vi "verifySignatureExample.vi"(8 "error in (no error)":errorcluster, 10 "verifySignatureRequestid":dbl) -> (0 "error out":errorcluster, 2 "verifySignatureResponse":T3)   [LabVIEW 2014]
uses:
  Type Defs/verifySignatureResponse.ctl
  Type Defs/generateIntegersRequest.ctl
  Type Defs/generateSignedIntegersResponse.ctl
  Sub Vi's/verifySignatures/verifySignatureIntegers.vi
  Random JSON API.lvlib
panel:
  in  "Force verification failure":bool
  out "Response":T1={"result"={"random"={"method"="", "hashedApiKey"="", "n"=0, "min"=0, "max"=0, "replacement"=TRUE, "base"=10, "data"=[], "completionTime"="", "serialNumber"=0}, "signature"="", "bitsUsed"=0, "bitsLeft"=0, "requestsLeft"=0, "advisoryDelay"=0}, "id"=0.0} {"result"."random"."base" items=["2"=2, "8"=8, "10"=10, "16"=16]}
  in  "Parameters":T2={"params"={"apiKey"="", "n"=0, "min"=0, "max"=0, "replacement"=TRUE, "base"=10}, "id"=0.0} {"params"."base" items=["2"=2, "8"=8, "10"=10, "16"=16]}
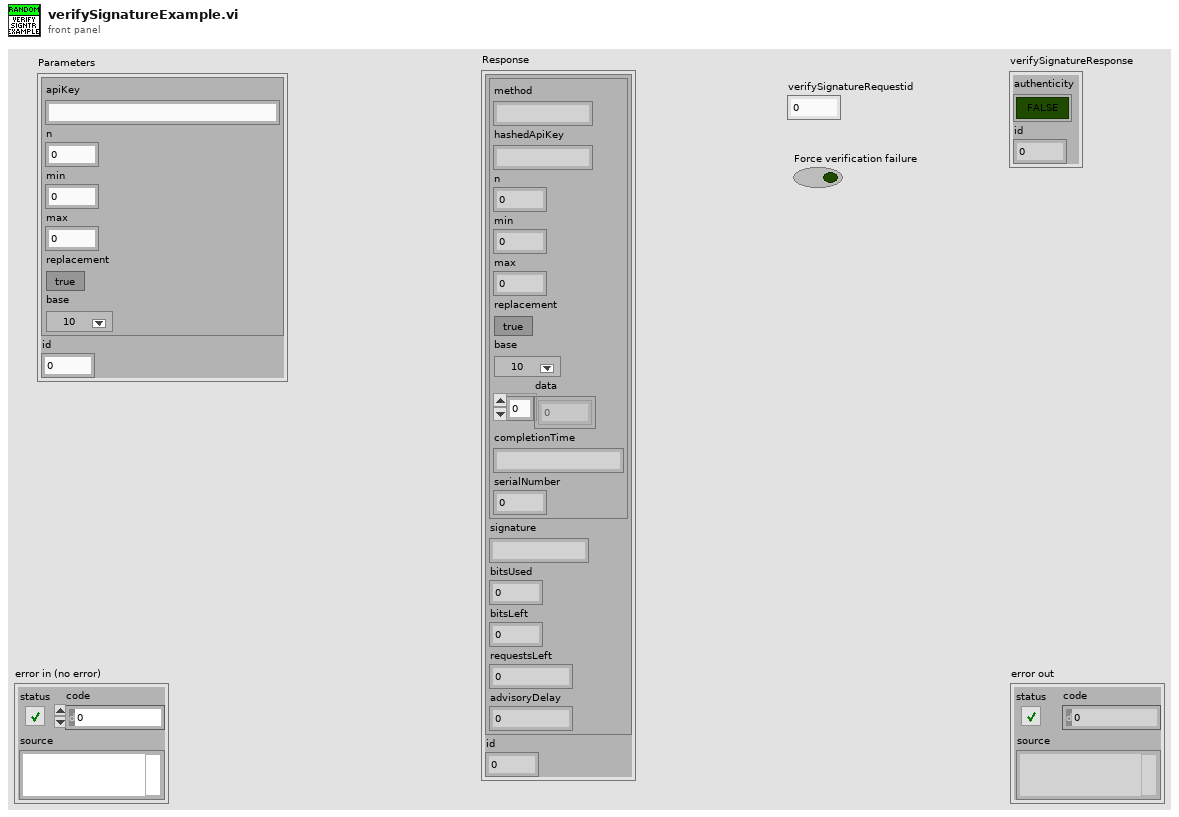
[diagram p1: front panel]
types:
  T1 = typedef "Random JSON API.lvlib/generateSignedIntegersResponse.ctl" = cluster{"result":cluster{"random":cluster{"method":string, "hashedApiKey":string, "n":i32, "min":i32, "max":i32, "replacement":bool, "base":i32, "data":i32[], "completionTime":string, "serialNumber":i32}, "signature":string, "bitsUsed":i32, "bitsLeft":i32, "requestsLeft":i32, "advisoryDelay":i32}, "id":dbl}
  T2 = typedef "Random JSON API.lvlib/generateIntegersRequest.ctl" = cluster{"params":cluster{"apiKey":string, "n":i32, "min":i32, "max":i32, "replacement":bool, "base":i32}, "id":dbl}
  T3 = typedef "Random JSON API.lvlib/verifySignatureResponse.ctl" = cluster{"authenticity":bool, "id":dbl}
  T4 = cluster{"method":string, "hashedApiKey":string, "n":i32, "min":i32, "max":i32, "replacement":bool, "base":i32, "data":i32[], "completionTime":string, "serialNumber":i32}
  T5 = cluster{"random":cluster{"method":string, "hashedApiKey":string, "n":i32, "min":i32, "max":i32, "replacement":bool, "base":i32, "data":i32[], "completionTime":string, "serialNumber":i32}, "signature":string, "verifySignatureRequestid":dbl}
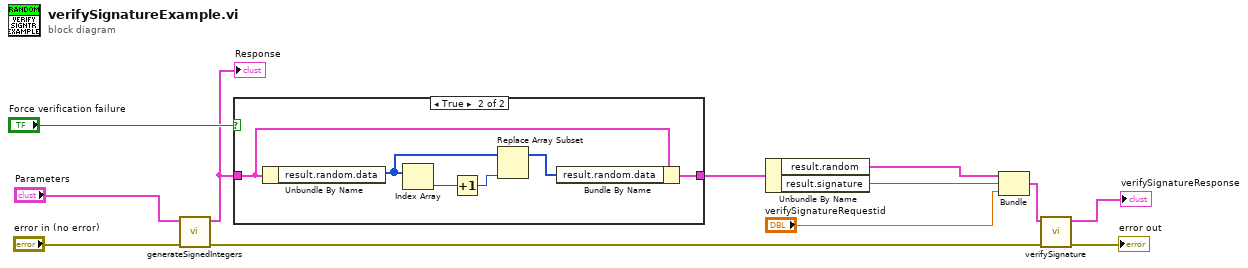
[diagram p0: block diagram]
diagram:
  n1 = call "generateSignedIntegers.vi"("error in (no error)"="error in (no error)", "Parameters"="Parameters") -> ("error out"=w12:errorcluster, "Response"=w1:T1)  [unwired: 7 in, 1 out]
  "Response" <- w1
  n2 = case shown="True" "Force verification failure" {
    tunnel: w1 -> [w13 w19]
    tunnel: [w13 w18] -> w3
    frame False {
    }
    frame True {
      n3 = Unbundle By Name(w19) -> ("result.random.data"=w16:i32[])
      n4 = Index Array(array=w16) -> (element=w17:i32)  [unwired: 1 in]
      n5 = Increment(x=w17) -> (x+1=w14:i32)
      n6 = Replace Array Subset(array=w16, new element=w14) -> (w15:i32[])  [unwired: 1 in]
      n7 = Bundle By Name(cluster=w19, "result.random.data"=w15) -> (w18:T1)
    }
  }
  n8 = Unbundle By Name(w3) -> ("result.random"=w6:T4, "result.signature"=w5:string)
  n9 = Bundle("random"=w6, "signature"=w5, "verifySignatureRequestid"="verifySignatureRequestid") -> (w7:T5)  [unwired: 1 in]
  n10 = call-poly "verifySignature.vi"("error in (no error)"=w12, "Request"=w7) -> ("error out"=→"error out":errorcluster, "Response"=→"verifySignatureResponse":T3)  [unwired: 7 in, 1 out]
